vi "Data Message_ASCII.vi"(7 "Parent Index":i32=-1, 8 "error in":errorcluster, 10 "Data":string, 11 "SECS-II Class in":refnum<class "SECS-II Class.lvclass">) -> (0 "error out":errorcluster, 3 "SECS-II Class out":refnum<class "SECS-II Class.lvclass">)   [LabVIEW 2020, in "SECS Communication.lvlib" / "SECS-II Class.lvclass"]
uses:
  SECS-II Class.lvclass
  SECS-II Class.lvclass/SECS-II Class.ctl
  Message Data.ctl
  Data Item Format.ctl
  Format Code.ctl
  Data To Variant_ASCII.vi
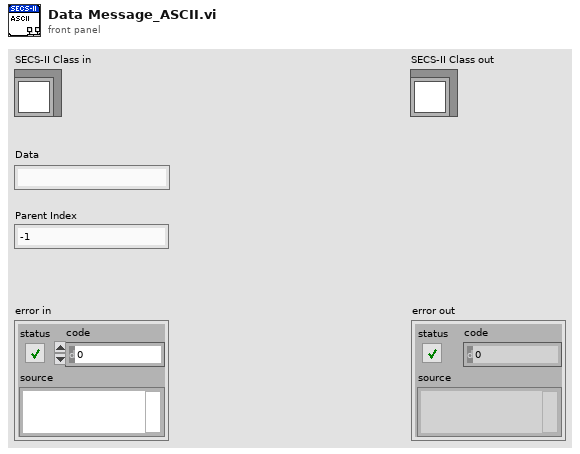
[diagram p1: front panel]
types:
  T1 = typedef "SECS Communication.lvlib/SECS-II Class.lvclass/Data Item Format.ctl" = enum16{"Data Type", "Value"}
  T2 = typedef "SECS Communication.lvlib/SECS-II Class.lvclass/Format Code.ctl" = enum16{"L", "A", "B", "Boolean", "J", "I1", "I2", "I4", "I8", "U1", "U2", "U4", "U8", "F4", "F8", "Char"}
  T3 = typedef "SECS Communication.lvlib/SECS-II Class.lvclass/Message Data.ctl" = cluster{"Index":i32, "Data Item Format":T1, "Format Code":T2, "Parent Index":i32, "Child Index":i32[], "Data":variant}
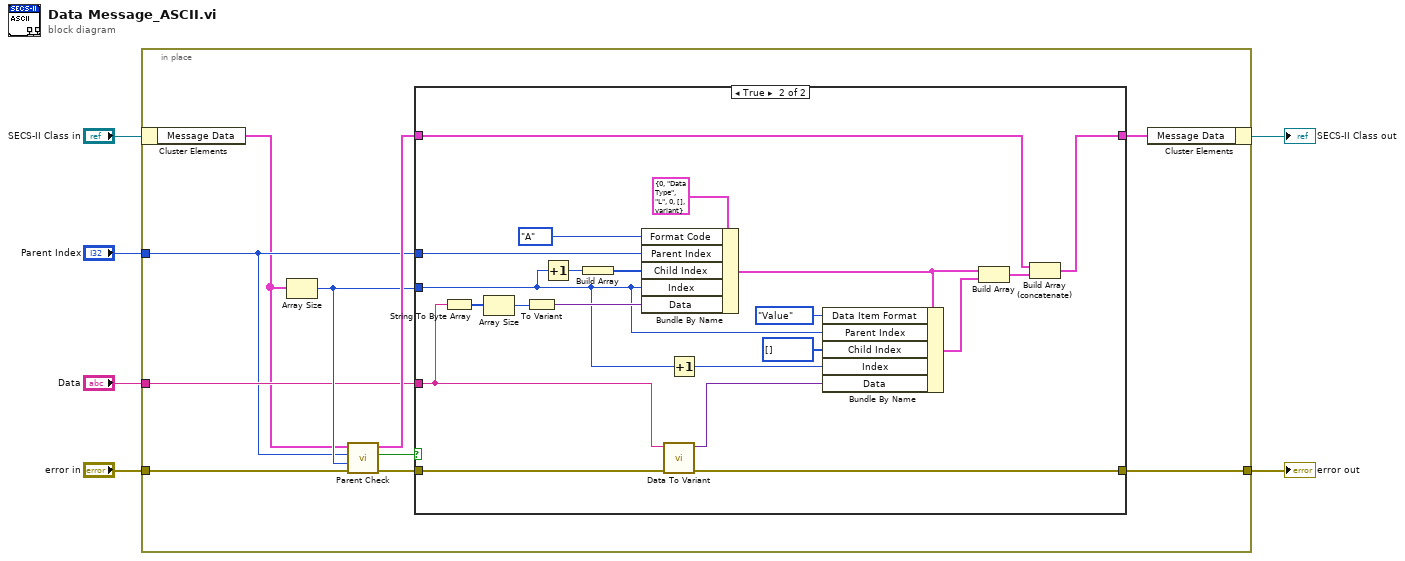
[diagram p0: block diagram]
diagram:
  n1 = in-place {
    in-place-border: "error in" -> [w7]
    in-place-border: [w12] -> w5
    in-place-border: "Data" -> [w11]
    in-place-border: "Parent Index" -> [w10]
    n2 = in-place-cluster #1("SECS-II Class in") -> ("Message Data"=w9:T3[])
    n3 = Array Size(array=w9) -> (size(s)=w13:i32)
    n4 = call "Parent Check.vi"("error in"=w7, "Message Index"=w13, "Parent Index"=w10, "Message Data In"=w9) -> ("error out"=w15:errorcluster, "OK?"=w16:bool, "Message Data Out"=w14:T3[])  [unwired: 5 in]
    n5 = case shown="True" w16 {
      tunnel: w15 -> [w17 w22]
      tunnel: w14 -> [w18 w26]
      tunnel: [w18 w25] -> w8
      tunnel: w10 -> [_ w32]
      tunnel: w13 -> [_ w24]
      tunnel: w11 -> [_ w21]
      tunnel: [w17 w19] -> w12
      frame False {
      }
      frame True {
        n6 = String To Byte Array(string=w21) -> (unsigned byte array=w23:u8[])
        n7 = Array Size(array=w23) -> (size(s)=w35:i32)
        n8 = To Variant(anything=w35) -> (Variant=w34:variant)
        n9 = Increment(x=w24) -> (x+1=w37:i32)
        n10 = Build Array(w37) -> (w36:i32[])
        n11 = Bundle By Name(cluster=T3 {"Index"=0, "Data Item Format"=enum."Data Type", "Format Code"=enum."L", "Parent Index"=0, "Child Index"=[], "Data"=variant} ("Message Data"), "Format Code"=Format_Code."A", "Parent Index"=w32, "Child Index"=w36, "Index"=w24, "Data"=w34) -> (w29:T3)
        n12 = call-poly "Data To Variant.vi"("error in (no error)"=w22, "Data"=w21) -> ("error out"=w19:errorcluster, "Variant"=w20:variant)  [unwired: 8 in]
        n13 = Increment(x=w24) -> (x+1=w30:i32)
        n14 = Bundle By Name(cluster=w29, "Data Item Format"=Data_Item_Format."Value", "Parent Index"=w24, "Child Index"=i32[] [], "Index"=w30, "Data"=w20) -> (w28:T3)
        n15 = Build Array(w29, w28) -> (w27:T3[])
        n16 = Build Array (concatenate)(w26, w27) -> (w25:T3[])
      }
    }
    n17 = in-place-cluster #1("Message Data"=w8) -> (→"SECS-II Class out":refnum<class "SECS-II Class.lvclass">)
  }
  "error out" <- w5
